vi "emi_Create Unknown Type Error.vi"(0 "Anything":variant, 11 "error IO":errorcluster) -> (15 "error out":errorcluster)   [LabVIEW 2011]
doc: "Creates teh Unknown data type error for the type library vis"
uses:
  <vilib>/Utility/VariantDataType/VariantType.lvlib
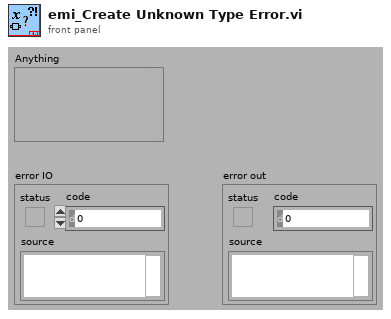
[diagram p1: front panel]
types:
  T1 = typedef "VariantType.lvlib/Type.ctl" = enum8{"Invalid Type", "Void", "I8", "I16", "I32", "I64", "U8", "U16", "U32", "U64", "Single Float", "Double Float", "Extended Float", "Single Complex", "Double Complex", "Extended Complex", "Enum U8", "Enum U16", "Enum U32", "Enum U64", "Single Float With Unit", "Double Float With Unit", "Extended Float With Unit", "Single Complex with Unit", "Double Complex with Unit", "Extended Complex with Unit", "Boolean", "String", "Path", "Picture", "Tag", "Array", "Cluster", "Variant", "LV Variant", "Waveform", "Timestamp", "Digital Waveform", "Digital Data", "ExpressData", "Refnum", "External Data", "VI", "Poly VI", "LabVIEW Class Instance", "Fixed Point"}
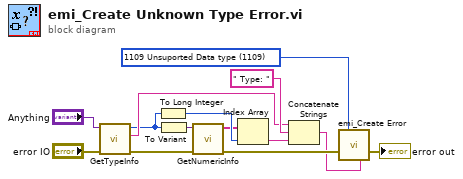
[diagram p0: block diagram]
diagram:
  w2 = 1109 items=["0 No Error"=0, "1 Invalid input parameter"=1, "6 Generic file IO "=6, "7 File not Found"=7, "35 Generic Pring Error"=35, "37 Device not Found"=37, "39 Device Unit Error"=39, "40 Could fot Open Device"=40, "42 Generic Error"=42, "52 Unknown Message"=52, "98 Bad File type"=98, "99 Bad File Version"=99, "100 Bad Data in File"=100, "1018 Unspecefied Error"=1018, "1041 Incorrect Password"=1041, "1043 Feature not in this version"=1043, "1109 Unsuported Data type"=1109] ("Error Code")
  n1 = call <vilib>:"GetTypeInfo.vi"("error in (no error)"="error IO", "Variant"="Anything") -> ("error out"=w7:errorcluster, "Name"=w13:string, "Type Enum"=w9:T1)  [unwired: 5 in, 2 out]
  n2 = To Long Integer(number=w9) -> (32bit integer=w11:i32)
  n3 = To Variant(anything=w9) -> (Variant=w8:variant)
  n4 = call <vilib>:"GetNumericInfo.vi"("error in (no error)"=w7, "Variant"=w8) -> ("error out"=w4:errorcluster, "EnumNames"=w10:string[])  [unwired: 6 in, 2 out]
  n5 = Index Array(array=w10, index=w11) -> (element=w12:string)
  n6 = Concatenate Strings(w13, " Type: " ("string"), w12) -> (w1:string)
  n7 = call "emi_Create Error.vi"("Error Code"=w2, "error in (no error)"=w4, "Append String(\"\")"=w1) -> ("error out"=→"error out":errorcluster)  [unwired: 12 in]
